vi "Write DAQmxTask dict-mem.vi"(8 "error in (no error)":errorcluster, 9 "Task name":T2, 10 "cluster":T1, 11 "Control in":refnum<class "Control.lvclass">) -> (0 "error out":errorcluster, 3 "Control out":refnum<class "Control.lvclass">)   [LabVIEW 2015]
uses:
  Control.lvclass
  dependecies/ControlsVIs/Clusters-def/list-of-DAQmx-tasks.ctl
  DAQmxTasks/DAQmxTask.lvclass
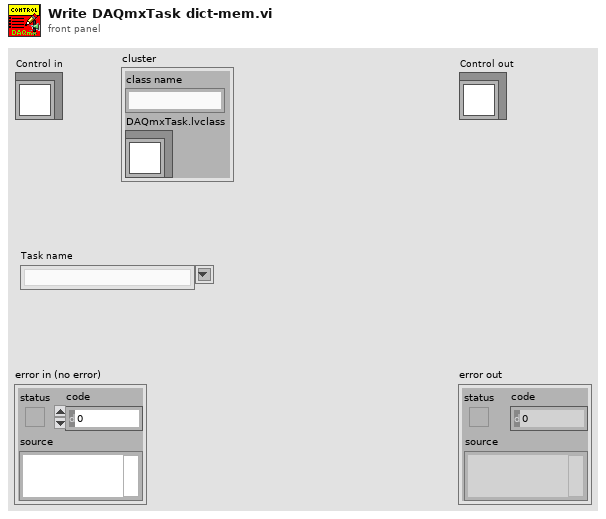
[diagram p1: front panel]
types:
  T1 = cluster{"class name":string, "DAQmxTask.lvclass":refnum<class "DAQmxTask.lvclass">}
  T2 = typedef "list-of-DAQmx-tasks.ctl" = string
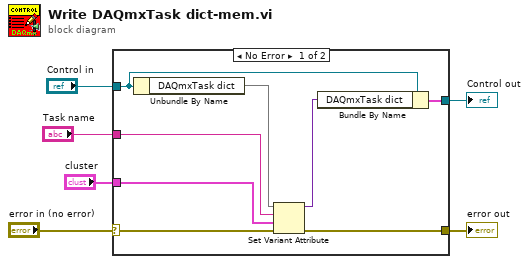
[diagram p0: block diagram]
diagram:
  n1 = case shown="No Error" "error in (no error)" {
    selector: "error in (no error)" -> [w9 w15]
    tunnel: [w8 w15] -> w5
    tunnel: [w14 w16] -> w3
    tunnel: "Control in" -> [w13 w16]
    tunnel: "Task name" -> [w10 _]
    tunnel: "cluster" -> [w7 _]
    frame No Error {
      n2 = Unbundle By Name(w13) -> ("DAQmxTask dict"=w12)
      n3 = Set Variant Attribute(Variant=w12, name=w10, value=w7, error in=w9) -> (Variant out=w11:variant, error out=w8:errorcluster)  [unwired: 1 out]
      n4 = Bundle By Name(cluster=w13, "DAQmxTask dict"=w11) -> (w14:cluster{})
    }
    frame Error {
    }
  }
  "error out" <- w5
  "Control out" <- w3
